vi "Get Memory Buffer Size.vi"(11 "Buffer in":refnum<class "Memory Buffer.lvclass">) -> (2 "buffer size":u64, 3 "Buffer out":refnum<class "Memory Buffer.lvclass">)   [LabVIEW 2017, in "Data Sharing Framework Engine.lvlib" / "Memory Buffer.lvclass"]
uses:
  Memory Buffer.lvclass
  Memory Buffer.lvclass/Memory Buffer.ctl
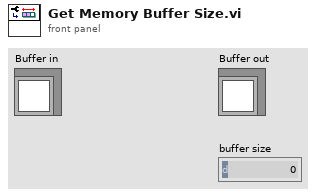
[diagram p1: front panel]
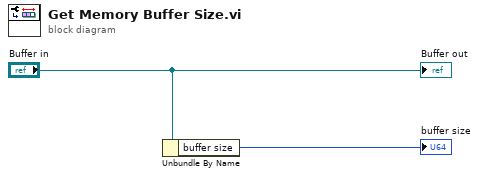
[diagram p0: block diagram]
diagram:
  n1 = Unbundle By Name("Buffer in") -> ("buffer size"=→"buffer size":u64)
  "Buffer out" <- "Buffer in"
